vi "FXP_L_ye_Bend_u_singleAxis_32bit.vi"(7 "NS":u8=5, 8 "U(k): ux":fxp<+/-,32,5>, 11 "Y(k): x":fxp<+/-,32,5>) -> (0 "yd_est":fxp<+/-,32,5>, 2 "outputValid":bool)   [LabVIEW 2019]
uses:
  <vilib>/Platform/TimedLoop/XDataNode/timing_clust.ctl
  <vilib>/Platform/TimedLoop/XDataNode/nitl_modes.ctl
  <vilib>/Platform/TimedLoop/XDataNode/wakeup.ctl
  typeDefs/Lz_bram.ctl
  typeDefs/Bz_bram.ctl
  typeDefs/x_vec_bram.ctl
  <vilib>/rvi/Emulation/niFpgaSctlEmulationGetInTimedLoop.vi
  <vilib>/rvi/Emulation/niFpgaEmulationReportErrorSimple.vi
  <vilib>/rvi/Emulation/niFpgaGetClockAttributes.vi
  <vilib>/rvi/Emulation/niFpgaCriticalErrorInLSC.vi
  <vilib>/rvi/DataTransferAndStorage/Container/Common/niFpgaContainerExecOnDevCompGetState.vi
  <vilib>/rvi/Emulation/niFpgaEmulationIsFPGAContextNoSignature.vi
  <vilib>/rvi/DataTransferAndStorage/Container/Common/niFpgaContainerGetUniqueNameForEmu.vi
  <vilib>/rvi/Emulation/niFpgaProcessEmulError.vi
  <vilib>/rvi/errors/nirviReportUnexpectedCaseInternalError (U32).vi
  <vilib>/rvi/Memory/Memory_Emulation/niFpgaMemoryEmulationCacheClearOnFirstRun.vi
  <vilib>/rvi/Memory/Memory_Emulation/nirvimemoryEmulationManagerCache_MakeExclusive.vi
  <vilib>/rvi/Memory/Memory_Emulation/niFpgaMemoryEmulationValidateCache.vi
  <vilib>/rvi/Memory/Memory_Emulation/nirvimemoryEmulationManagerCache_InsertValue.vi
  <vilib>/Utility/error.llb/Clear Errors.vi
  <vilib>/rvi/Memory/Memory_Emulation/nirvimemoryEmulationManagerCache_ReleaseExclusive.vi
  <vilib>/rvi/Memory/Memory_Emulation/nirvimemoryEmulationManagerCache_GetValue.vi
  <vilib>/rvi/Memory/Memory_Emulation/nirvimemoryEmulationManagerCache_SetValue.vi
  <vilib>/rvi/Emulation/niFpgaSctlEmulationResourceMgr.vi
  <vilib>/Platform/TimedLoop/XDataNode/XDataNode.xnode
  <vilib>/rvi/DataTransferAndStorage/Container/XNode/niFpgaContainer.xnode
  <vilib>/rvi/Memory/Memory_Emulation/niFpgaMemoryEmulationRefIn.vi
  <vilib>/rvi/FXPMathLib/FxpAdd/XNode/nifxpmath_Add.xnode
  <vilib>/rvi/DataTransferAndStorage/Register/Emulation/niFpgaRegisterEmulation.vi
  <vilib>/Platform/TimedLoop/XDataNode/XDNodeRunTimeDep.lvlib
  <vilib>/rvi/FXPMathLib/sim/FxpSim.dll
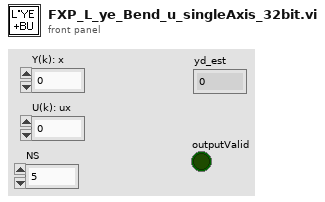
[diagram p1: front panel]
types:
  T1 = typedef "XDNodeRunTimeDep.lvlib/timing_clust.ctl" = cluster{"Expected End [f-1]":u64, "Actual End [f-1]":u64, "Finished Late? [f-1]":bool, "Expected End [i-1]":u64, "Actual End [i-1]":u64, "Finished Late? [i-1]":bool, "Expected Start [i]":u64, "Actual Start [i]":u64, "Expected Start [f]":u64, "Actual Start [f]":u64, "Source Name":string, "Structure Name":string, "Period":i64, "Deadline":i64, "Offset":i64, "Start":i64, "Priority":i32, "Timeout":i32, "Mode":T2, "Wakeup Reason":T3, "Error":errorcluster, "Source Type":string, "Secondary Source Type":string, "Global End Time":u64, "Global Start Time":u64, "Frame Duration":u64, "Iteration Duration":u64, "Assigned CPU":i32, "I/O Scan Engine Mode":u32}
  T2 = typedef "XDNodeRunTimeDep.lvlib/nitl_modes.ctl" = enum32{"No Change", "Process missed periods, maintain original phase", "Discard missed periods, maintain original phase", "Process missed periods, ignore original phase", "Discard missed periods, ignore original phase"}
  T3 = typedef "XDNodeRunTimeDep.lvlib/wakeup.ctl" = enum32{"Normal", "Aborted", "Asynchronous wakeup", "Timing source error", "Timed loop error", "Timeout"}
  T4 = typedef "x_vec_bram.ctl" = refnum<k21>
  T5 = typedef "Bz_bram.ctl" = refnum<k21>
  T6 = typedef "Lz_bram.ctl" = refnum<k21>
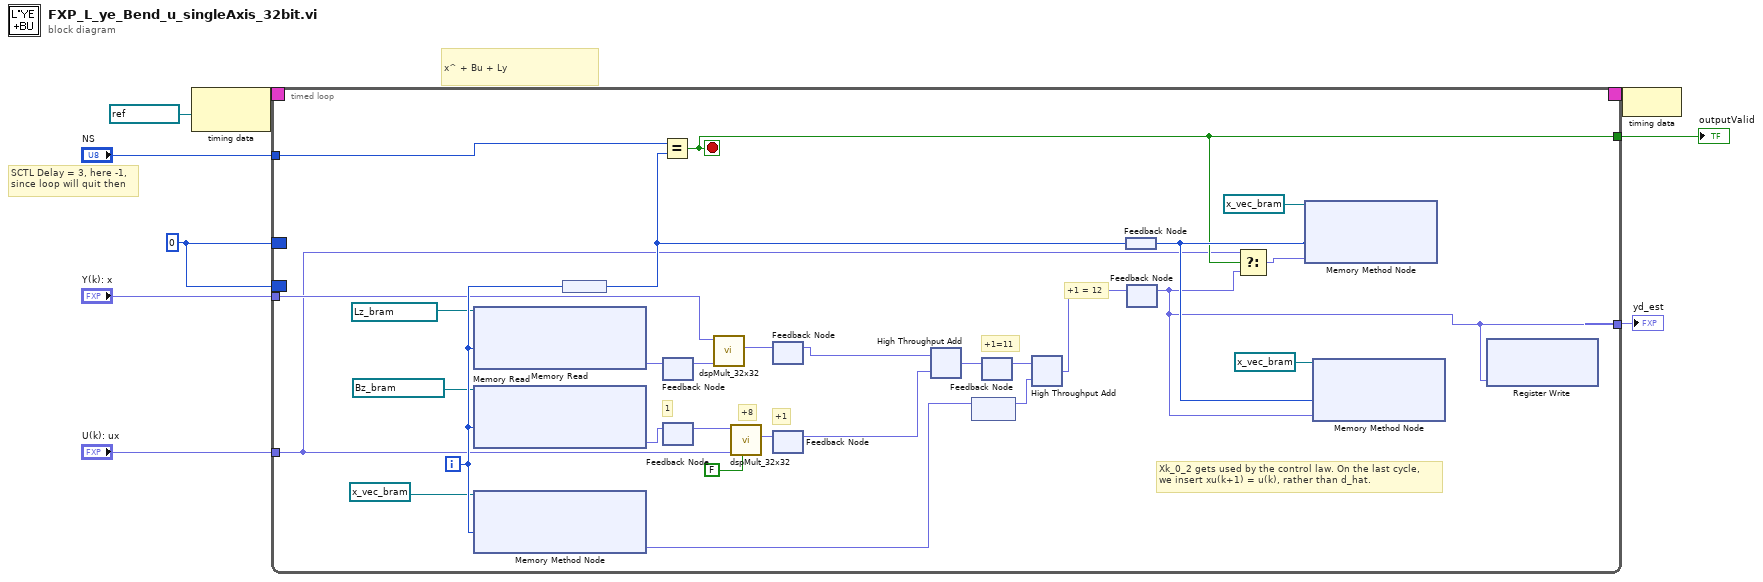
[diagram p0: block diagram]
diagram:
  w4 = 0
  # "x^ + Bu + Ly"
  # "SCTL Delay = 3, here -1,\nsince loop will quit then"
  n1 = node-c288(refnum<k21> "80MHz" ("Source Name")) -> (w9:T1)
  n2 = timed-loop {
    timing: w9 -> [_]
    timing-out: [_] -> w8
    tunnel: "NS" -> [w37]
    border: w4 -> [_]
    tunnel: [w12] -> w6
    border: w4 -> [_]
    tunnel: "Y(k): x" -> [w23]
    tunnel: "U(k): ux" -> [w10]
    tunnel: [w11] -> w3
    i -> [w24]
    stop <- w12 stop-if-true
    # "+1 = 12"
    # "+1=11"
    # "+1"
    # "+8"
    # "1"
    # "Xk_0_2 gets used by the control law. On the last cycle,\nwe insert xu(k+1) = u(k), rather than d_hat."
    n3 = xnode ("Memory Read")("Address"=w24, "Memory In"=T6 "L_FXP_col1" ("Memory")) -> ("Data"=w34:fxp<+/-,32,3>)  [unwired: 1 out]
    n4 = xnode ("Memory Read")("Address"=w24, "Memory In"=T5 "Bz_FXP_col1" ("Memory")) -> ("Data"=w36:fxp<+/-,32,3>)  [unwired: 1 out]
    n5 = xnode ("Memory Method Node")("Address"=w24, "Memory In"=T4 "xk_1_0" ("Memory")) -> ("Data"=w35:fxp<+/-,32,6>)  [unwired: 1 out]
    n6 = feedback #1() -> (w30:i32)
    n7 = feedback-in #1(w24) -> ()
    n8 = Equal?(x=w37, y=w30) -> (x = y?=w12:bool)
    n9 = feedback #2() -> (w28:fxp<+/-,32,3>)  [unwired: 1 in]
    n10 = feedback-in #2(w34) -> ()
    n11 = feedback #3() -> (w27:fxp<+/-,32,3>)  [unwired: 1 in]
    n12 = feedback-in #3(w36) -> ()
    n13 = call "dspMult_32x32.vi"("b"=w28, "a"=w23) -> ("p"=w29:fxp<+/-,64,10>)  [unwired: 9 in]
    n14 = call "dspMult_32x32.vi"("sclr"=FALSE ("input valid"), "b"=w10, "a"=w27) -> ("p"=w26:fxp<+/-,64,10>)  [unwired: 8 in]
    n15 = feedback #4() -> (w16:fxp<+/-,64,10>)  [unwired: 1 in]
    n16 = feedback-in #4(w29) -> ()
    n17 = feedback #5() -> (w15:fxp<+/-,64,10>)  [unwired: 1 in]
    n18 = feedback-in #5(w26) -> ()
    n19 = xnode ("High Throughput Add")("x"=w16, "y"=w15) -> ("x+y"=w33:fxp<+/-,32,8>)
    n20 = feedback #6() -> (w31:fxp<+/-,32,6>)  [unwired: 1 in]
    n21 = feedback-in #6(w35) -> ()
    n22 = feedback #7() -> (w32:fxp<+/-,32,8>)  [unwired: 1 in]
    n23 = feedback-in #7(w33) -> ()
    n24 = xnode ("High Throughput Add")("x"=w32, "y"=w31) -> ("x+y"=w22:fxp<+/-,32,6>)
    n25 = feedback #8() -> (w14:i32)
    n26 = feedback-in #8(w30) -> ()
    n27 = feedback #9() -> (w11:fxp<+/-,32,6>)  [unwired: 1 in]
    n28 = feedback-in #9(w22) -> ()
    n29 = Select(t=w10, s=w12, f=w11) -> (s? t:f=w13:fxp<+/-,33,6>)
    n30 = xnode ("Memory Method Node")("Address"=w14, "Data"=w13, "Memory In"=T4 "xk_0_2" ("Memory")) -> ()  [unwired: 1 out]
    n31 = xnode ("Memory Method Node")("Address"=w14, "Data"=w11, "Memory In"=T4 "xk_0_1" ("Memory")) -> ()  [unwired: 1 out]
    n32 = xnode "Register Write"("Data"=w11) -> ()  [unwired: 1 in, 1 out]
  }
  "outputValid" <- w6
  "yd_est" <- w3
  n33 = node-c288(w8) -> ()
